vi "ZE_Recorder_CreateTDMS.vi"(5 "Header Cluster":T1={"Project"="", "Operator ID"="", "Description"="Measurement Description: "}, 7 "Sampling Rate [Hz]":dbl, 8 "error in (no error)":errorcluster, 10 "Channel Array":T2 {"Terminal" items=["Default"=-1, "RSE"=10083, "NRSE"=10078, "Differential"=10106, "Pseudodifferential"=12529]}, 11 "TDMS Path":path) -> (0 "error out":errorcluster, 2 "Name Array":string[](array[string]), 3 "TDMS Refnum out":refnum<k34>)   [LabVIEW 2025, in "ZE_Recorder.lvlib"]
doc: "ZE_Recorder_CreateTDMS.vi\n----------------------------------------------\nThe VI creates the TDMS and writes the channel properties to the file\n\nInputs:\n---------------------\n- error in (no error) : Cluster; \n- Range : DBL; \n- Channel Array : 1DArrayOfCluster; \n- TDMS Path : Path; \n\nOutputs:\n---------------------\n- error out : Cluster; \n- Name Array : 1DArrayOfString; \n- TDMS Refnum out : Refnum; \n\n----------------------------------------------\n03.06.2016\nZühlke Engineering AG\nCH-8952 Schlieren\nwww.zuehlke.com"
uses:
  ZE_Recorder.lvlib
  ZE_Recorder_ChannelCluster.ctl
  ChannelCluster.ctl
  ZE_Recorder_Units.ctl
  Temperature.ctl
  ZE_Recorder_Header.ctl
panel:
  # "Connector Pane"
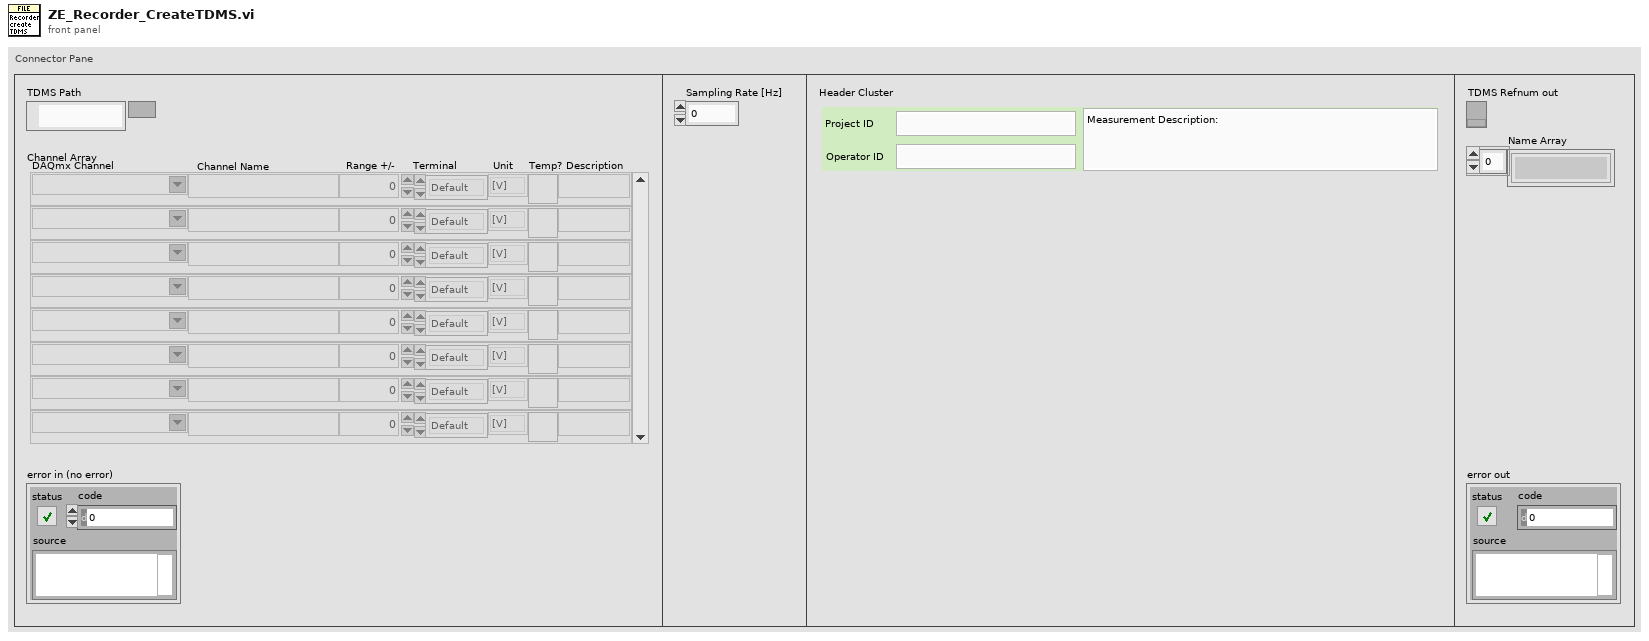
[diagram p1: front panel]
types:
  T1 = typedef "ZE_Recorder.lvlib/ZE_Recorder_Header.ctl" = cluster{"Project":string, "Operator ID":string, "Description":string}
  T2 = typedef "ZE_Recorder.lvlib/ZE_Recorder_ChannelCluster.ctl" = T3[]
  T3 = typedef "ZE_Recorder.lvlib/ChannelCluster.ctl" = cluster{"physical channel":tag, "channel name":string, "Range":dbl, "Terminal":i32, "Unit":T4, "isTemp":T5, "Description":string}
  T4 = typedef "ZE_Recorder.lvlib/ZE_Recorder_Units.ctl" = enum16{"[V]", "[A]", "[F]", "[H]", "[°C]", "[ml/s]", "[m/s]", "[bar]", "[%]", "[N]", "[?]"}
  T5 = typedef "ZE_Recorder.lvlib/Temperature.ctl" = bool
  T6 = enum16{"open", "open or create", "create or replace", "create", "open (read-only)"}
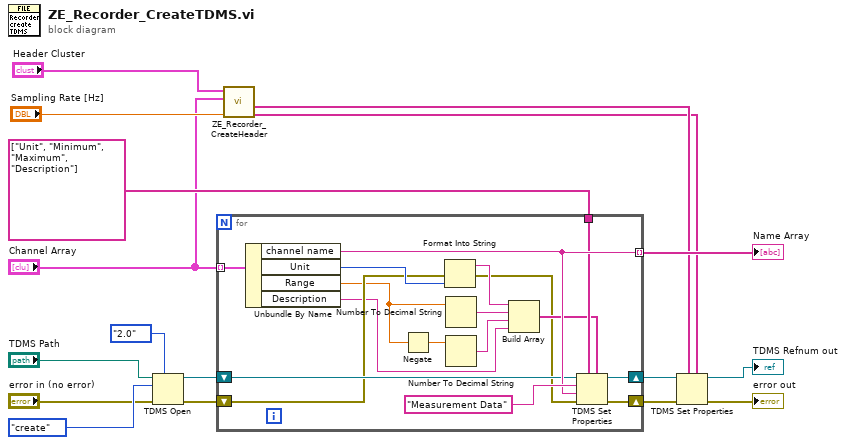
[diagram p0: block diagram]
diagram:
  n1 = TDMS Open(7:enum16{"1.0", "2.0"}."2.0" ("file format version (2.0)"), 8:"error in (no error)", 10:T6."create" ("operation (0:open)"), 11:"TDMS Path") -> (0:w10:errorcluster, 3:w11:refnum<k34>)  [unwired: 3 in]
  n2 = for {
    tunnel: "Channel Array" -> [w34] mode=indexing
    tunnel: [w32] -> w17 mode=indexing
    shift-right: [w31] -> w6
    shift-left: w10 -> [w26]
    shift-right: [w29] -> w5
    shift-left: w11 -> [w30]
    tunnel: string[] ["Unit", "Minimum", "Maximum", "Description"] ("property names") -> [w28]
    n3 = Unbundle By Name(w34) -> ("channel name"=w32:string, "Unit"=w27:T4, "Range"=w20:dbl, "Description"=w18:string)
    n4 = Negate(x=w20) -> (-x=w25:dbl)
    n5 = Format Into String(error in=w26, w27) -> (resulting string=w24:string, error out=w21:errorcluster)  [unwired: 2 in]
    n6 = Number To Decimal String(number=w20) -> (decimal integer string=w23:string)  [unwired: 1 in]
    n7 = Number To Decimal String(number=w25) -> (decimal integer string=w19:string)  [unwired: 1 in]
    n8 = Build Array(w24, w23, w19, w18) -> (w22:string[])
    n9 = TDMS Set Properties(5:w22, 7:w28, 8:w21, 9:w32, 10:"Measurement Data" ("group name"), 11:w30) -> (0:w31:errorcluster, 3:w29:refnum<k34>)  [unwired: 2 out]
  }
  "Name Array" <- w17
  n10 = call "ZE_Recorder_CreateHeader.vi"("Sampling Rate"="Sampling Rate [Hz]", "Channel Array"="Channel Array", "Header Cluster"="Header Cluster") -> ("TDMS propValues"=w1:string[], "TDMS properties"=w2:string[])  [unwired: 6 in, 1 out]
  n11 = TDMS Set Properties(5:w1, 7:w2, 8:w6, 11:w5) -> (0:→"error out":errorcluster, 3:→"TDMS Refnum out":refnum<k34>)  [unwired: 2 in, 2 out]
